vi "data to graphs.vi"(10 "data in":T2(array[cluster])) -> (1 "graph coincidences":cluster{timestamp[], u32[]}[](array[cluster]), 2 "graph singles":cluster{timestamp[], u32[]}[](array[cluster]))   [LabVIEW 2015]
doc: "Group graph data according to their tpye: singles or coindent counters."
uses:
  <instrlib>/Tausand AB1000/Public/Controls/counters4ch.ctl
  <instrlib>/Tausand AB1000/Tausand AB1000.lvlib
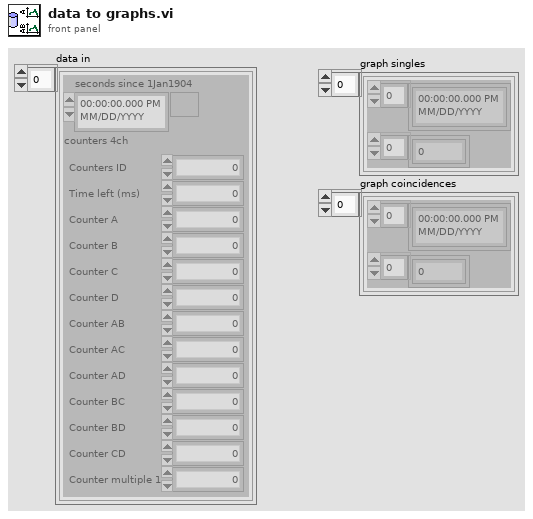
[diagram p1: front panel]
types:
  T1 = typedef "Tausand AB1000.lvlib/counters4ch.ctl" = cluster{"counter_A":u32, "counter_B":u32, "counter_C":u32, "counter_D":u32, "counter_AB":u32, "counter_AC":u32, "counter_AD":u32, "counter_BC":u32, "counter_BD":u32, "counter_CD":u32, "counter_multiple_1":u32, "counters_ID":u32, "time_left":u32}
  T2 = cluster{"seconds since 1Jan1904":timestamp, "counters 4ch":T1}[]
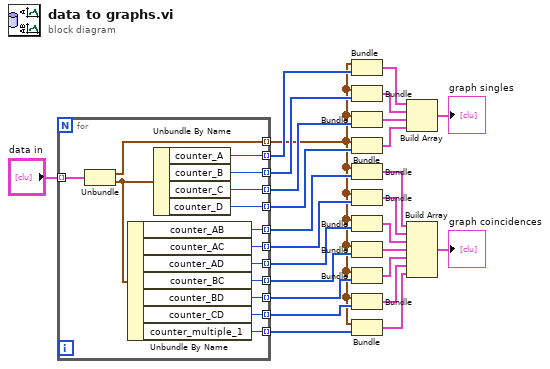
[diagram p0: block diagram]
diagram:
  n1 = for {
    tunnel: "data in" -> [w40] mode=indexing
    tunnel: [w39] -> w2 mode=indexing
    tunnel: [w38] -> w20 mode=indexing
    tunnel: [w37] -> w21 mode=indexing
    tunnel: [w36] -> w22 mode=indexing
    tunnel: [w35] -> w23 mode=indexing
    tunnel: [w33] -> w16 mode=indexing
    tunnel: [w32] -> w15 mode=indexing
    tunnel: [w31] -> w14 mode=indexing
    tunnel: [w30] -> w13 mode=indexing
    tunnel: [w29] -> w12 mode=indexing
    tunnel: [w28] -> w11 mode=indexing
    tunnel: [w27] -> w3 mode=indexing
    n2 = Unbundle(w40) -> ("seconds since 1Jan1904"=w39:timestamp, "counters 4ch"=w34:T1)
    n3 = Unbundle By Name(w34) -> ("counter_AB"=w33:u32, "counter_AC"=w32:u32, "counter_AD"=w31:u32, "counter_BC"=w30:u32, "counter_BD"=w29:u32, "counter_CD"=w28:u32, "counter_multiple_1"=w27:u32)
    n4 = Unbundle By Name(w34) -> ("counter_A"=w38:u32, "counter_B"=w37:u32, "counter_C"=w36:u32, "counter_D"=w35:u32)
  }
  n5 = Bundle(w2, w20) -> (w19:cluster{timestamp[], u32[]})  [unwired: 1 in]
  n6 = Bundle(w2, w21) -> (w24:cluster{timestamp[], u32[]})  [unwired: 1 in]
  n7 = Bundle(w2, w22) -> (w25:cluster{timestamp[], u32[]})  [unwired: 1 in]
  n8 = Bundle(w2, w23) -> (w26:cluster{timestamp[], u32[]})  [unwired: 1 in]
  n9 = Bundle(w2, w16) -> (w10:cluster{timestamp[], u32[]})  [unwired: 1 in]
  n10 = Bundle(w2, w15) -> (w9:cluster{timestamp[], u32[]})  [unwired: 1 in]
  n11 = Bundle(w2, w14) -> (w8:cluster{timestamp[], u32[]})  [unwired: 1 in]
  n12 = Bundle(w2, w13) -> (w7:cluster{timestamp[], u32[]})  [unwired: 1 in]
  n13 = Bundle(w2, w12) -> (w6:cluster{timestamp[], u32[]})  [unwired: 1 in]
  n14 = Bundle(w2, w11) -> (w5:cluster{timestamp[], u32[]})  [unwired: 1 in]
  n15 = Bundle(w2, w3) -> (w1:cluster{timestamp[], u32[]})  [unwired: 1 in]
  n16 = Build Array(w19, w24, w25, w26) -> (→"graph singles":cluster{timestamp[], u32[]}[])
  n17 = Build Array(w10, w9, w8, w7, w6, w5, w1) -> (→"graph coincidences":cluster{timestamp[], u32[]}[])
